vi "test - Idea Validation.vi"(8 "error in (no error)":errorcluster, 11 "TestCase in":refnum<class "csm-ini-variable-addon.lvclass">) -> (0 "error out":errorcluster, 3 "TestCase out":refnum<class "csm-ini-variable-addon.lvclass">)   [LabVIEW 2017, in "csm-ini-variable-addon.lvclass"]
uses:
  csm-ini-variable-addon.lvclass
  INI-Static-Variable-Support/INI-Static-Variable-Support.lvlib
  <userlib>/_NEVSTOP/Communicable State Machine(CSM)/Communicable State Machine.lvlib
panel:
  out "x > 0?":bool
  out "section string":string
  out "script":string
  out "Contained Variables":string[](array[string])
  out "String out":string
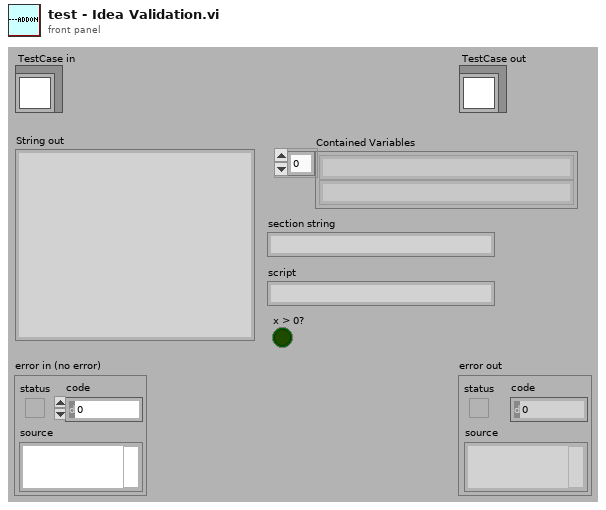
[diagram p1: front panel]
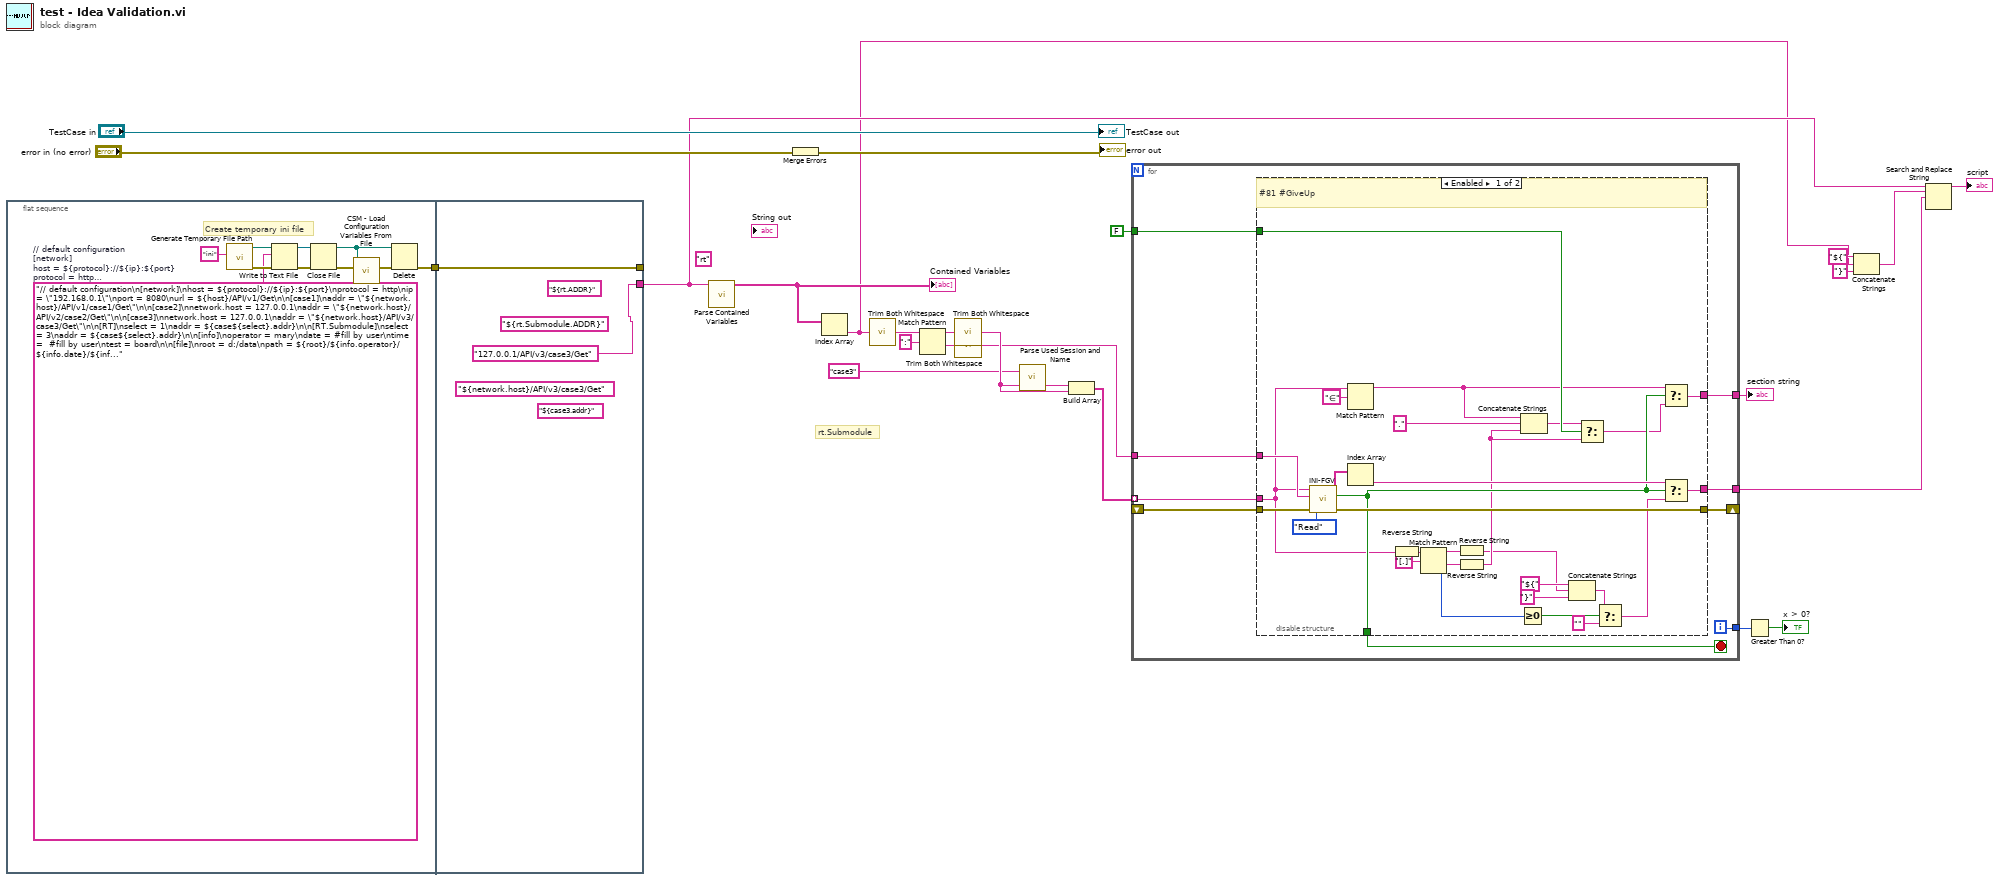
[diagram p0: block diagram]
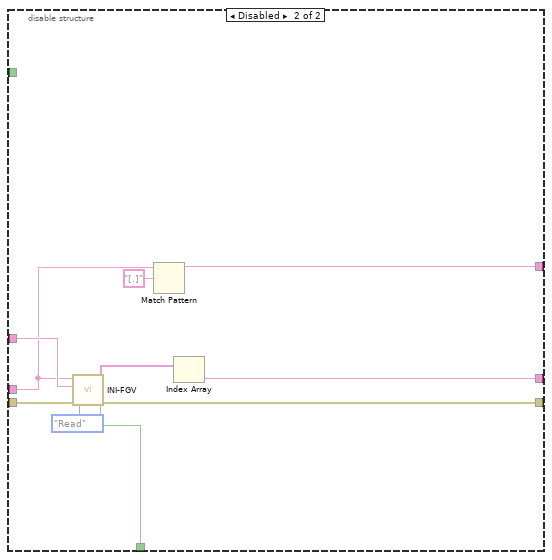
[diagram p2: hidden frame]
diagram:
  (unwired) "rt" ("Section Name(\"\" as Default)")
  # "rt.Submodule"
  n1 = flat-sequence {
    tunnel: [w35] -> w22
    tunnel: [w37] -> _
    tunnel: w22 -> [w37]
    tunnel: ["127.0.0.1/API/v3/case3/Get" ("String in")] -> w3
    frame #0 {
      w28 = "// default configuration\n[network]\nhost = ${protocol}://${ip}:${port}\nprotocol = http\nip = \"192.168.0.1\"\nport = 8080\nurl = ${host}/API/v1/Get\n\n[case1]\naddr = \"${network.host}/API/v1/case1/Get\"\n\n[case2]\nnetwork.host = 127.0.0.1\naddr = \"${network.host}/API/v2/case2/Get\"\n\n[case3]\nnetwork.host = 127.0.0.1\naddr = \"${network.host}/API/v3/case3/Get\"\n\n[RT]\nselect = 1\naddr = ${case${select}.addr}\n\n[RT.Submodule]\nselect = 3\naddr = ${case${select}.addr}\n\n[info]\noperator = mary\ndate = #fill by user\ntime =  #fill by user\ntest = board\n\n[file]\nroot = d:/data\npath = ${root}/${info.operator}/${info.date}/${info.test}${info.time}.tdms"  # // default configuration [network] host = ${protocol}://${ip}:${port} protocol = http ip = "192.168.0.1" port = 8080 url = ${host}/API/v1/Get  [case1] addr = "${network.host}/API/v1/case1/Get"  [case2] network.host = 127.0.0.1 addr = "${network.host}/API/v2/case2/Get"  [case3] network.host = 127.0.0.1 addr = "${network.host}/API/v3/case3/Get"  [RT] select = 1 addr = ${case${select}.addr}  [RT.Submodule] select = 3 addr = ${case${select}.addr}  [info] operator = mary date = #fill by user time =  #fill by user test = board  [file] root = d:/data path = ${root}/${info.operator}/${info.date}/${info.test}${info.time}.tdms
      # "Create temporary ini file"
      n2 = call <vilib>:"Generate Temporary File Path.vi"("Temporary File Extension (tmp)"="ini") -> ("error out"=w34:errorcluster, "Unique Temporary File Path"=w31:path)  [unwired: 9 in]
      n3 = Write to Text File(file (use dialog)=w31, text=w28, error in=w34) -> (refnum out=w30:refnum<file>, error out=w32:errorcluster)  [unwired: 1 in, 1 out]
      n4 = Close File(refnum=w30, error in=w32) -> (path=w26:path, error out=w29:errorcluster)
      n5 = call "CSM - Load Configuration Variables From File.vi"("error in (no error)"=w29, "Path"=w26) -> ("error out"=w27:errorcluster)  [unwired: 7 in]
      n6 = Delete(path (use dialog)=w26, error in=w27) -> (error out=w35:errorcluster)  [unwired: 3 in, 2 out]
    }
    frame #1 {
      (unwired) "${case3.addr}" ("String in")
      (unwired) "${network.host}/API/v3/case3/Get" ("String in")
      (unwired) "${rt.Submodule.ADDR}" ("String in")
      (unwired) "${rt.ADDR}" ("String in")
    }
  }
  n7 = call "Parse Contained Variables.vi"("String"=w3) -> ("Contained Variables"=w15:string[])  [unwired: 10 in]
  "Contained Variables" <- w15
  n8 = Merge Errors("error in (no error)") -> (→"error out":errorcluster)
  n9 = Index Array(array=w15) -> (element=w1:string)  [unwired: 1 in]
  n10 = call <userlib>:"Trim Both Whitespace.vi"("string"=w1) -> ("trimmed string"=w18:string)  [unwired: 1 in]
  n11 = Match Pattern(string=w18, regular expression=":") -> (before substring=w20:string, after substring=w19:string)  [unwired: 1 in, 2 out]
  n12 = call <userlib>:"Trim Both Whitespace.vi"("string"=w20) -> ("trimmed string"=w17:string)  [unwired: 1 in]
  n13 = call <userlib>:"Trim Both Whitespace.vi"("string"=w19) -> ("trimmed string"=w11:string)  [unwired: 1 in]
  n14 = call "Parse Used Session and Name.vi"("name"=w17, "Section Name(\"\" as Default)"="case3" ("Section Name(\"\" as Default)")) -> ("used name"=w16:string)  [unwired: 1 in]
  n15 = Build Array(w16, w17) -> (w12:string[])
  n16 = for {
    tunnel: w11 -> [w46]
    tunnel: [w40] -> w10
    tunnel: [w45] -> w2
    tunnel: w12 -> [w41] mode=indexing
    shift-right: [w44] -> _
    shift-left: _ -> [w42]
    tunnel: FALSE ("Last empty section?") -> [w38]
    tunnel: [w39] -> w9
    i -> [w39]
    stop <- w43 stop-if-true
    n17 = disable-structure shown="Enabled" {
      disable-tunnel: w46 -> [w75 w85]
      disable-tunnel: [w68 w82] -> w45
      disable-tunnel: [w72 w81] -> w44
      disable-tunnel: [w60 w80] -> w43
      disable-tunnel: w42 -> [w71 w79]
      disable-tunnel: w41 -> [w47 w78]
      disable-tunnel: [w59 w77] -> w40
      disable-tunnel: w38 -> [w55 _]
      frame Enabled {
        # "#81 #GiveUp"
        n18 = call "INI-FGV.vi"("Enum"=enum16{"Read", "Write", "Sync"}."Read", "error IN"=w71, ">> Default Value >>"=w75, ">> Variable Name >>"=w47) -> ("error out"=w72:errorcluster, "Key?"=w60:bool, "Array"=w74:string[])  [unwired: 4 in, 1 out]
        n19 = Match Pattern(string=w47, regular expression="∈" ("search string")) -> (before substring=w48:string)  [unwired: 1 in, 3 out]
        n20 = Index Array(array=w74) -> (element=w69:string)  [unwired: 1 in]
        n21 = Reverse String(1:w47) -> (0:w52:string)
        n22 = Match Pattern(string=w52, regular expression="[.]") -> (before substring=w51:string, after substring=w57:string, offset past match=w67:i32)  [unwired: 1 in, 1 out]
        n23 = Reverse String(1:w51) -> (0:w49:string)
        n24 = Reverse String(1:w57) -> (0:w50:string)
        n25 = Greater Or Equal To 0?(x=w67) -> (x >= 0?=w66:bool)
        n26 = Concatenate Strings(w48, "." ("string"), w50) -> (w54:string)
        n27 = Concatenate Strings("${" ("regular expression"), w49, "}" ("regular expression")) -> (w65:string)
        n28 = Select(t=w54, s=w55, f=w50) -> (s? t:f=w53:string)
        n29 = Select(t=w65, s=w66, f="") -> (s? t:f=w64:string)
        n30 = Select(t=w48, s=w60, f=w53) -> (s? t:f=w59:string)
        n31 = Select(t=w69, s=w60, f=w64) -> (s? t:f=w68:string)
      }
      frame Disabled {
        n32 = call "INI-FGV.vi"("Enum"=enum16{"Read", "Write", "Sync"}."Read", "error IN"=w79, ">> Default Value >>"=w85, ">> Variable Name >>"=w78) -> ("error out"=w81:errorcluster, "Key?"=w80:bool, "Array"=w84:string[])  [unwired: 4 in, 1 out]
        n33 = Match Pattern(string=w78, regular expression="[.]") -> (before substring=w77:string)  [unwired: 1 in, 3 out]
        n34 = Index Array(array=w84) -> (element=w82:string)  [unwired: 1 in]
      }
    }
  }
  "section string" <- w10
  n35 = Greater Than 0?(x=w9) -> (x > 0?=→"x > 0?":bool)
  n36 = Concatenate Strings("${" ("regular expression"), w1, "}" ("regular expression")) -> (w5:string)
  n37 = Search and Replace String(input string=w3, search string=w5, replace string=w2) -> (result string=→"script":string)  [unwired: 5 in, 3 out]
  "TestCase out" <- "TestCase in"
